vi "client.vi"() -> ()   [LabVIEW 2018]
uses:
  Global_Variable/Global.vi
panel:
  in  "设备信息":T1={"设备名称"="芯轴分总成磨合台", "操作人员"="", "设备状态"=enum."设备离线", "附加信息"=""}
  in  "服务器关闭":string="服务器VI关闭了连接。"
  in  "停止":bool
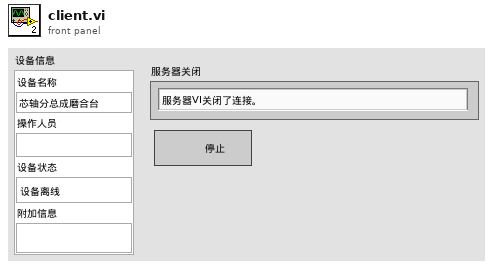
[diagram p1: front panel]
types:
  T1 = cluster{"设备名称":string, "操作人员":string, "设备状态":enum16{"设备离线", "设备正常", "设备缺料", "设备故障", "质量报警"}, "附加信息":string}
  T2 = enum32{"Invalid", "Standard", "Closed", "Hidden", "Minimized", "Maximized"}
  T3 = cluster{"设备名称":bool, "操作人员":bool, "设备状态":bool, "附加信息":bool}
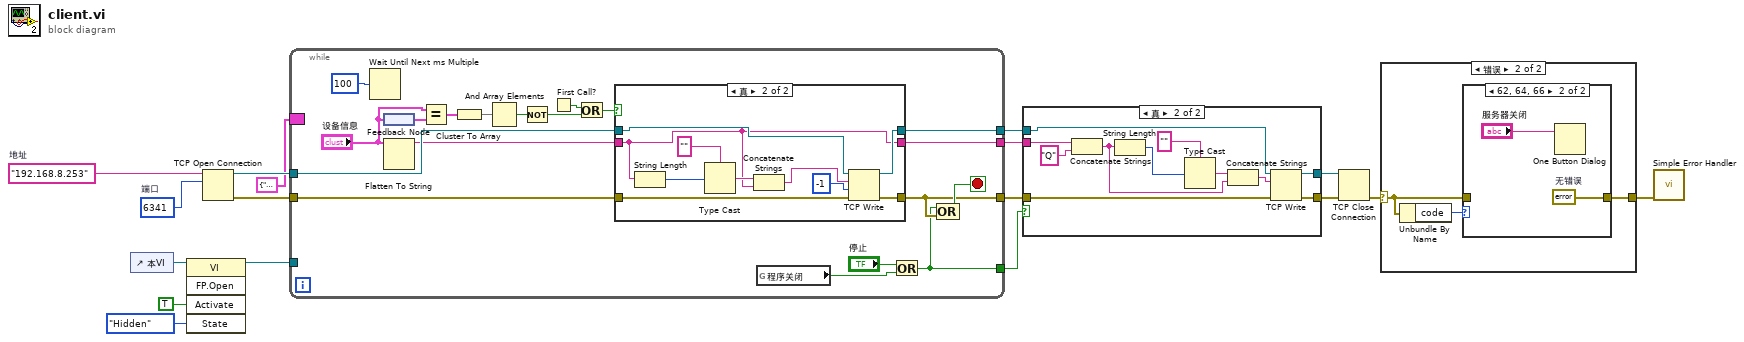
[diagram p0: block diagram]
diagram:
  w16 = u16 6341  # 端口
  w17 = "192.168.8.253"  # 地址
  n1 = control-ref of="本VI"() -> (w2:refnum<vi>)
  n2 = invoke class="VI" method="FP.Open"(reference=w2, "Activate"=TRUE ("激活？"), "State"=T2."Hidden" ("状态")) -> (reference out=w1:refnum<vi>)  [unwired: 2 in, 4 out]
  n3 = TCP Open Connection(address=w17, remote port or service name=w16) -> (connection ID=w15:refnum<k5>, error out=w14:errorcluster)  [unwired: 1 in, 2 out]
  n4 = while {
    tunnel: [w19] -> w9
    tunnel: [w34] -> w13
    tunnel: [w31] -> w11
    tunnel: w14 -> [w35]
    tunnel: w15 -> [w36]
    tunnel: [w24] -> w6
    border: T1 {"设备名称"="", "操作人员"="", "设备状态"=enum."设备正常", "附加信息"=""} ("设备信息") -> [_]
    tunnel: w1 -> [_]
    stop <- w33 stop-if-true
    n5 = Wait Until Next ms Multiple(millisecond multiple=u32 100 ("毫秒倍数")) -> ()  [unwired: 1 out]
    n6 = feedback-in #1("设备信息") -> ()
    n7 = feedback #1() -> (w28:T1)
    n8 = Flatten To String(anything="设备信息") -> (data string=w25:string)  [unwired: 3 in, 2 out]
    n9 = Equal?(x="设备信息", y=w28) -> (x = y?=w27:T3)
    n10 = Cluster To Array(cluster=w27) -> (array=w26:bool[])
    n11 = And Array Elements(Boolean array=w26) -> (logical AND=w23:bool)
    n12 = Not(x=w23) -> (.not. x?=w20:bool)
    n13 = First Call?() -> (First Call?: T/F=w21:bool)
    n14 = Or(x=w21, y=w20) -> (x .or. y?=w22:bool)
    n15 = case shown="真" w22 {
      tunnel: w36 -> [w39 w49]
      tunnel: w35 -> [w38 w48]
      tunnel: [w39 w47] -> w34
      tunnel: [w38 w46] -> w31
      tunnel: w25 -> [w37 w40]
      tunnel: [w37 w40] -> w24
      frame False {
      }
      frame True {
        n16 = String Length(string=w40) -> (length=w44:i32)
        n17 = Type Cast(type="", x=w44) -> (*(type *) &x=w42:string)
        n18 = Concatenate Strings(w42, w40) -> (w41:string)
        n19 = TCP Write(connection ID=w49, data in=w41, error in (no error)=w48, 9:-1) -> (connection ID out=w47:refnum<k5>, error out=w46:errorcluster)  [unwired: 1 out]
      }
    }
    n20 = global read "Global.vi" "程序关闭"() -> (w18:bool)
    n21 = Or(x="停止", y=w18) -> (x .or. y?=w19:bool)
    n22 = Compound Arithmetic op=OR ("复合运算")(w19, w31) -> (w33:bool)
  }
  n23 = case shown="真" w9 {
    tunnel: w13 -> [w51 w62]
    tunnel: [w51 w60] -> w12
    tunnel: w11 -> [w50 w61]
    tunnel: [w50 w59] -> w10
    tunnel: w6 -> [_ w57]
    frame False {
    }
    frame True {
      n24 = Concatenate Strings(w57, "Q") -> (w53:string)
      n25 = String Length(string=w53) -> (length=w56:i32)
      n26 = Type Cast(type="", x=w56) -> (*(type *) &x=w54:string)
      n27 = Concatenate Strings(w54, w53) -> (w52:string)
      n28 = TCP Write(connection ID=w62, data in=w52, error in (no error)=w61) -> (connection ID out=w60:refnum<k5>, error out=w59:errorcluster)  [unwired: 2 out]
    }
  }
  n29 = TCP Close Connection(connection ID=w12, error in (no error)=w10) -> (error out=w8:errorcluster)  [unwired: 2 out]
  n30 = case shown="错误" w8 {
    selector: w8 -> [w63 w65]
    tunnel: [w63 w64] -> w7
    frame No Error {
    }
    frame Error {
      n31 = Unbundle By Name(w65) -> ("code"=w66:i32)
      n32 = case shown="62, 64, 66" w66 {
        tunnel: w65 -> [w67 _]
        tunnel: [w67 w69] -> w64
        frame Default {
        }
        frame 62, 64, 66 {
          w69 = errorcluster {"status"=FALSE, "code"=0, "source"=""}  # 无错误
          n33 = One Button Dialog(message="服务器关闭") -> ()  [unwired: 1 in, 1 out]
        }
      }
    }
  }
  n34 = call <vilib>:"Simple Error Handler.vi"("error in (no error)"=w7) -> ()  [unwired: 1 in, 8 out]
